vi "MakeQNErrorCluster.vi"(4 "File Empty?":bool, 6 "Errer Cluster in":T3, 8 "TabControl in":refnum<vi>, 9 "Number Cluster in":T4, 10 "# of Errors":i32, 11 "Log":T2={"Sent"="", "Reply"="", "MethodName"="", "success"=FALSE, "XML Direction 1"="", "XML Direction 2"="", "VI Name"="", "close reference"={"status"=FALSE, "code"=0, "source"=""}, "release queue"={"status"=FALSE, "code"=0, "source"=""}, "release notification"={"status"=FALSE, "code"=0, "source"=""}, "varaiant to data"={"status"=FALSE, "code"=0, "source"=""}, "console error"={"status"=FALSE, "code"=0, "source"=""}, "Time Stamp"="", "ROS"={"topic port"=0, "Node"="", "topic"="", "type"="", "node port"=0, "error "={"status"=FALSE, "code"=0, "source"=""}, "Direction"=enum."Node", "Update (ms)"=1, "write queue"=1}}) -> (1 "Error Cluster out":T3, 2 "Number Cluster out":T4, 3 "servers qn":T5(array[cluster]))   [LabVIEW 2012]
uses:
  <userlib>/ROSforLV/ROS/Code/SubVIs/_ROSDirection.ctl
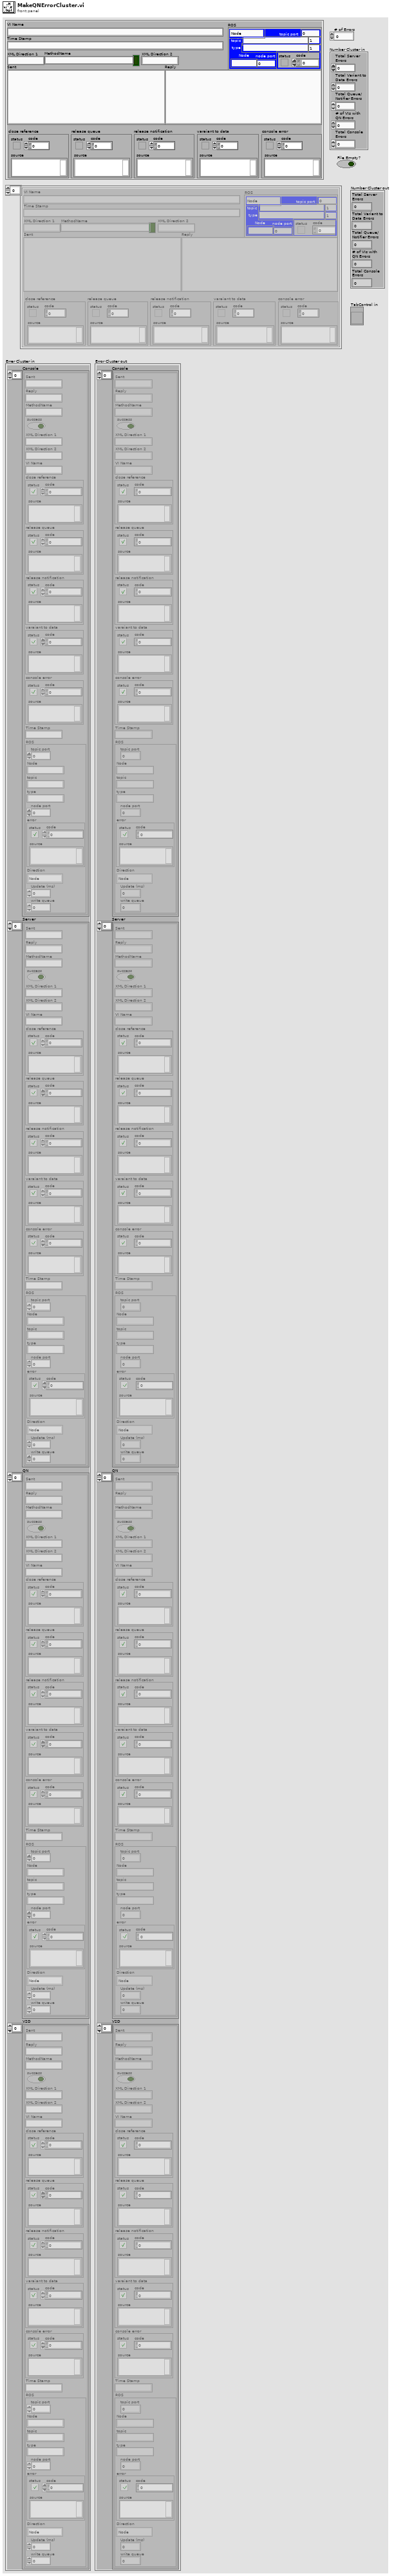
[diagram p1: front panel]
types:
  T1 = typedef "_ROSDirection.ctl" = enum16{"Node", "Publisher", "Subscriber", "Service Client"}
  T2 = cluster{"Sent":string, "Reply":string, "MethodName":string, "success":bool, "XML Direction 1":string, "XML Direction 2":string, "VI Name":string, "close reference":errorcluster, "release queue":errorcluster, "release notification":errorcluster, "varaiant to data":errorcluster, "console error":errorcluster, "Time Stamp":string, "ROS":cluster{"topic port":u16, "Node":string, "topic":string, "type":string, "node port":u32, "error ":errorcluster, "Direction":T1, "Update (ms)":u16, "write queue":u16}}
  T3 = cluster{"Console":cluster{"Sent":string, "Reply":string, "MethodName":string, "success":bool, "XML Direction 1":string, "XML Direction 2":string, "VI Name":string, "close reference":errorcluster, "release queue":errorcluster, "release notification":errorcluster, "varaiant to data":errorcluster, "console error":errorcluster, "Time Stamp":string, "ROS":cluster{"topic port":u16, "Node":string, "topic":string, "type":string, "node port":u32, "error ":errorcluster, "Direction":T1, "Update (ms)":u16, "write queue":u16}}[], "Server":cluster{"Sent":string, "Reply":string, "MethodName":string, "success":bool, "XML Direction 1":string, "XML Direction 2":string, "VI Name":string, "close reference":errorcluster, "release queue":errorcluster, "release notification":errorcluster, "varaiant to data":errorcluster, "console error":errorcluster, "Time Stamp":string, "ROS":cluster{"topic port":u16, "Node":string, "topic":string, "type":string, "node port":u32, "error ":errorcluster, "Direction":T1, "Update (ms)":u16, "write queue":u16}}[], "QN":cluster{"Sent":string, "Reply":string, "MethodName":string, "success":bool, "XML Direction 1":string, "XML Direction 2":string, "VI Name":string, "close reference":errorcluster, "release queue":errorcluster, "release notification":errorcluster, "varaiant to data":errorcluster, "console error":errorcluster, "Time Stamp":string, "ROS":cluster{"topic port":u16, "Node":string, "topic":string, "type":string, "node port":u32, "error ":errorcluster, "Direction":T1, "Update (ms)":u16, "write queue":u16}}[], "V2D":cluster{"Sent":string, "Reply":string, "MethodName":string, "success":bool, "XML Direction 1":string, "XML Direction 2":string, "VI Name":string, "close reference":errorcluster, "release queue":errorcluster, "release notification":errorcluster, "varaiant to data":errorcluster, "console error":errorcluster, "Time Stamp":string, "ROS":cluster{"topic port":u16, "Node":string, "topic":string, "type":string, "node port":u32, "error ":errorcluster, "Direction":T1, "Update (ms)":u16, "write queue":u16}}[]}
  T4 = cluster{"Total Server\nErrors":i32, "Total Variant to\nData Errors":i32, "Total Queue/\nNotifier Errors":i32, "# of VIs with\nQN Errors":i32, "Total Console\nErrors":i32}
  T5 = cluster{"Sent":string, "Reply":string, "MethodName":string, "success":bool, "XML Direction 1":string, "XML Direction 2":string, "VI Name":string, "close reference":errorcluster, "release queue":errorcluster, "release notification":errorcluster, "varaiant to data":errorcluster, "console error":errorcluster, "Time Stamp":string, "ROS":cluster{"topic port":u16, "Node":string, "topic":string, "type":string, "node port":u32, "error ":errorcluster, "Direction":T1, "Update (ms)":u16, "write queue":u16}}[]
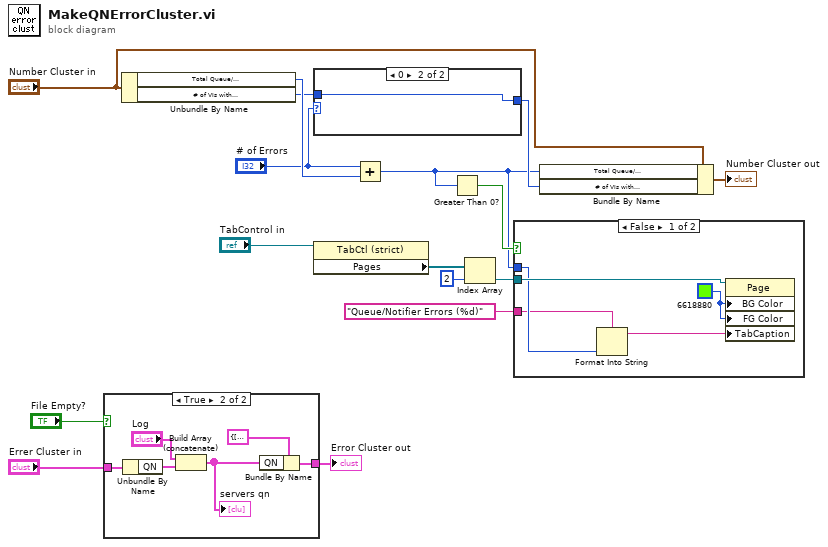
[diagram p0: block diagram]
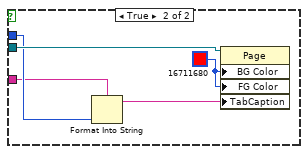
[diagram p3: hidden frame]
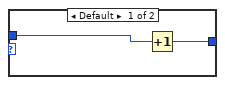
[diagram p4: hidden frame]
diagram:
  n1 = case shown="True" "File Empty?" {
    tunnel: [w17 w22] -> w11
    tunnel: "Errer Cluster in" -> [w17 w21]
    frame False {
    }
    frame True {
      n2 = Unbundle By Name(w21) -> ("QN"=w18:T5)
      n3 = Build Array (concatenate)("Log", w18) -> (w20:T5)
      "servers qn" <- w20
      n4 = Bundle By Name(cluster=T3 {"Console"=[], "Server"=[], "QN"=[], "V2D"=[]}, "QN"=w20) -> (w22:T3)
    }
  }
  "Error Cluster out" <- w11
  n5 = Unbundle By Name("Number Cluster in") -> ("Total Queue/\nNotifier Errors"=w16:i32, "# of VIs with\nQN Errors"=w14:i32)
  n6 = case shown="0" "# of Errors" {
    tunnel: w14 -> [w25 w26]
    tunnel: [w24 w26] -> w15
    frame Default {
      n7 = Increment(x=w25) -> (x+1=w24:i32)
    }
    frame 0 {
    }
  }
  n8 = property on="Property Node" class="TabCtl (strict)"(reference="TabControl in") -> ("Pages"=w7:refnum<vi>[])  [unwired: 1 in, 2 out]
  n9 = Add(x="# of Errors", y=w16) -> (x+y=w2:i32)
  n10 = Greater Than 0?(x=w2) -> (x > 0?=w9:bool)
  n11 = Index Array(array=w7, index=2) -> (element=w6:refnum<vi>)
  n12 = case shown="False" w9 {
    tunnel: w6 -> [w29 w36]
    tunnel: w2 -> [w28 w33]
    tunnel: "Queue/Notifier Errors (%d)" ("format string") -> [w27 w32]
    frame False {
      w31 = u32 6618880
      n13 = Format Into String(format string=w27, w28) -> (resulting string=w30:string)  [unwired: 2 in, 1 out]
      n14 = property on="Property Node" class="Page"(reference=w29, "BG Color"=w31, "FG Color"=w31, "TabCaption"=w30) -> ()  [unwired: 1 in, 2 out]
    }
    frame True {
      w35 = u32 16711680
      n15 = Format Into String(format string=w32, w33) -> (resulting string=w34:string)  [unwired: 2 in, 1 out]
      n16 = property on="Property Node" class="Page"(reference=w36, "BG Color"=w35, "FG Color"=w35, "TabCaption"=w34) -> ()  [unwired: 1 in, 2 out]
    }
  }
  n17 = Bundle By Name(cluster="Number Cluster in", "Total Queue/\nNotifier Errors"=w2, "# of VIs with\nQN Errors"=w15) -> (→"Number Cluster out":T4)
